vi "Auto Shift Control.vi"(11 "High/Low Gear Shift":bool) -> (3 "Low/High Gear Shift":enum16{"Off", "On", "Forward", "Reverse"}(ring))   [LabVIEW 2016]
uses:
  Global Variables/Low Gear Calibrations.vi
  Global Variables/Robot Status.vi
  Global Variables/Refnum Names.vi
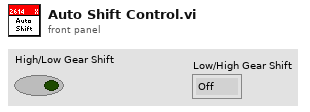
[diagram p1: front panel]
types:
  T1 = typedef "WPI_MotorControlDeviceRef.ctl" = cluster{"DeviceStatus":errorcluster, "Type":T2, "PWM":cluster{"PWM Channel":T3, "DeadBand":T4}, "CAN":cluster{"Device Number":u8, "SetOutput VI Ref":variant, "GetOutput VI Ref":variant, "Enable VI Ref":variant, "Disable VI Ref":variant, "Data":variant}, "Invert":bool}
  T2 = typedef "WPI_MotorControlType.ctl" = enum16{"PWM", "CAN"}
  T3 = typedef "FPGA_DIOPWMChannel.ctl" = enum8{"PWM 0", "PWM 1", "PWM 2", "PWM 3", "PWM 4", "PWM 5", "PWM 6", "PWM 7", "PWM 8", "PWM 9", "PWM MXP 0", "PWM MXP 1", "PWM MXP 2", "PWM MXP 3", "PWM MXP 4", "PWM MXP 5", "PWM MXP 6", "PWM MXP 7", "PWM MXP 8", "PWM MXP 9", "Invalid"}
  T4 = typedef "WPI_PWMDeadband.ctl" = cluster{"Name":string, "maxPositivePwm":i32, "minPositivePwm":i32, "centerPwm":i32, "maxNegativePwm":i32, "minNegativePwm":i32, "angularRange":u16}
  T5 = typedef "WPI_CANTalonSRX_GlobalStatus.ctl" = cluster{"Applied Throttle":dbl, "Module Enabled":bool, "CAN Error":errorcluster, "Closed Loop Error":dbl, "Forward Limit Switch Closed":bool, "Reverse Limit Switch Closed":bool, "Sensor Position":dbl, "Sensor Velocity":dbl, "Current":dbl, "Sticky Fault - Over Temp":bool, "Sticky Fault - Under Voltage":bool, "Sticky Fault - Forward Limit":bool, "Sticky Fault - Reverse Limit":bool, "Sticky Fault - Forward Soft Limit":bool, "Sticky Fault - Reverse Soft Limit":bool, "Brake is Enabled":bool, "Encoder Position":dbl, "Encoder Velocity":dbl, "Encoder Index Count":dbl, "Encoder A Pin State":bool, "Encoder B Pin State":bool, "Encoder Index Pin State":bool, "Analog In":dbl, "Analog In Velocity":dbl, "Temperature (C)":dbl, "Battery Voltage":dbl, "Control 5 Is Supported":bool, "Current Profile Slot Select":dbl, "Pos Div 8":bool, "Vel Div 4":bool, "Pulse Width Position":i32, "Pulse Width Velocity":i32, "Pulse Width Rise To Rise (us)":i32, "Pulse Width Rise To Fall (us)":i32, "Mot Prof Active Is Under Run":bool, "Mot Prof Active Has Under Run":bool, "Mot Prof Active Is Last":bool, "Mot Prof Active Velocity Only":bool, "Mot Prof Active Is Valid":bool, "Mot Prof Buffer Is Full":bool, "Mot Prof Active Profile Slot Select":i32, "Mot Prof NextID":i32, "Mot Prof Count":i32, "Mot Prof Active Velocity":dbl, "Mot Prof Active Position":dbl, "Mot Prof Output Enable":i32, "UsageFrame":u32, "Motion Magic Active Trajectory":cluster{"Velocity":dbl, "Position":dbl}}
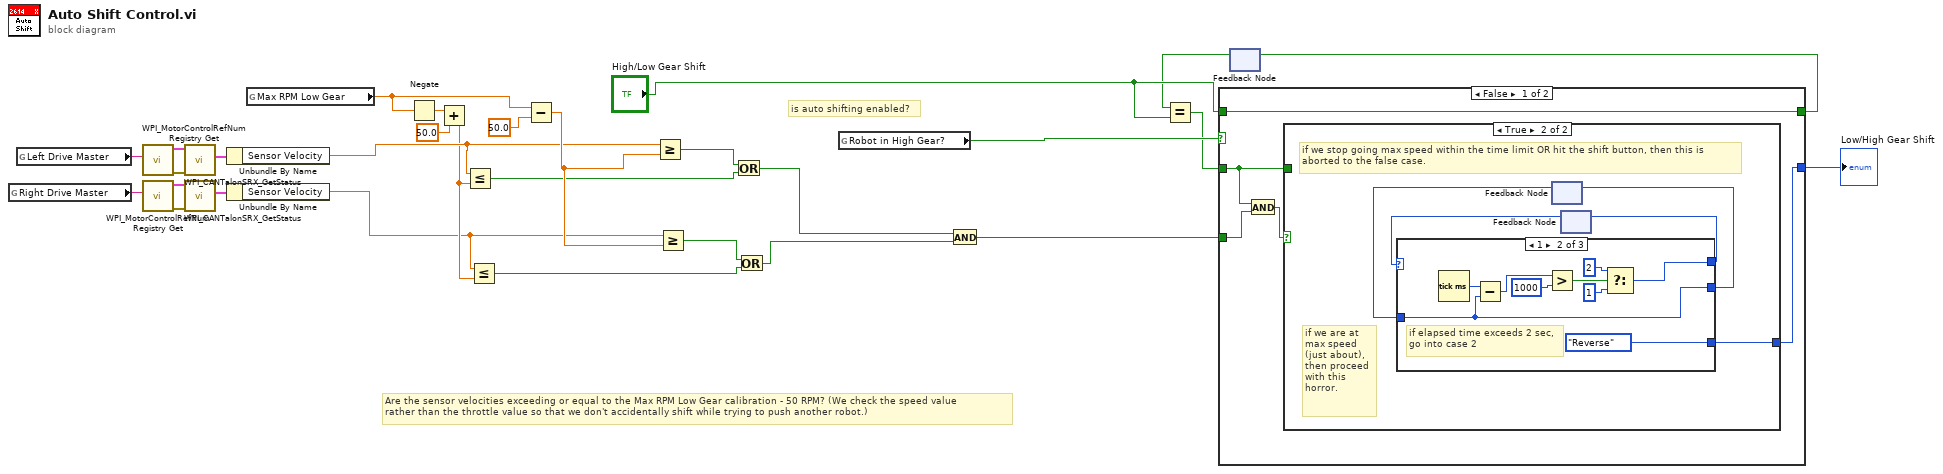
[diagram p0: block diagram]
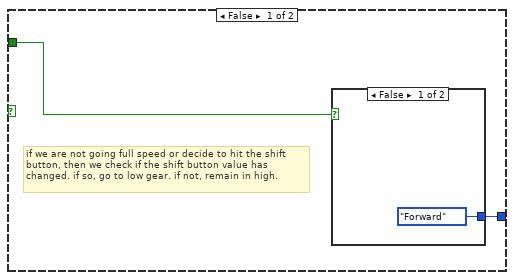
[diagram p2: hidden frame]
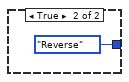
[diagram p3: hidden frame]
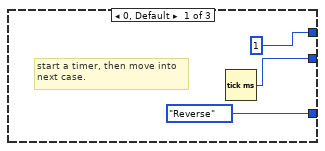
[diagram p4: hidden frame]
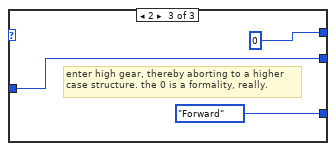
[diagram p5: hidden frame]
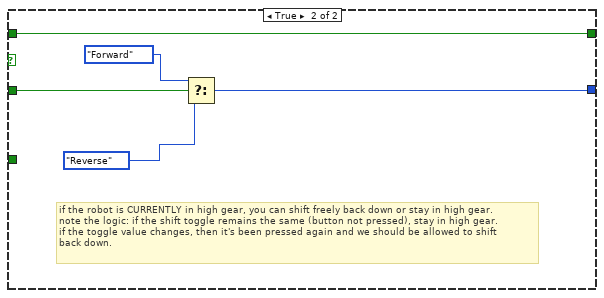
[diagram p6: hidden frame]
diagram:
  # "Are the sensor velocities exceeding or equal to the Max RPM Low Gear calibration - 50 RPM? (We check the speed value\nrather than the throttle value so that we don't accidentally shift while trying to push another robot.)"
  # "is auto shifting enabled?"
  n1 = global read "Refnum Names.vi" "Right Drive Master"() -> (w19:string)
  n2 = global read "Refnum Names.vi" "Left Drive Master"() -> (w22:string)
  n3 = call <vilib>:"WPI_MotorControlRefNum Registry Get.vi"("refnum name"=w22) -> ("error out"=w24:errorcluster, "MotorControlDevRef"=w23:T1)  [unwired: 9 in]
  n4 = call <vilib>:"WPI_MotorControlRefNum Registry Get.vi"("refnum name"=w19) -> ("error out"=w17:errorcluster, "MotorControlDevRef"=w18:T1)  [unwired: 9 in]
  n5 = call <vilib>:"WPI_CANTalonSRX_GetStatus.vi"("error in (no error)"=w24, "CAN Talon SRX Ref"=w23) -> ("Talon SRX Status"=w21:T5)  [unwired: 7 in, 2 out]
  n6 = call <vilib>:"WPI_CANTalonSRX_GetStatus.vi"("error in (no error)"=w17, "CAN Talon SRX Ref"=w18) -> ("Talon SRX Status"=w20:T5)  [unwired: 7 in, 2 out]
  n7 = Unbundle By Name(w21) -> ("Sensor Velocity"=w13:dbl)
  n8 = Unbundle By Name(w20) -> ("Sensor Velocity"=w11:dbl)
  n9 = global read "Low Gear Calibrations.vi" "Max RPM Low Gear"() -> (w16:dbl)
  n10 = Negate(x=w16) -> (-x=w14:dbl)
  n11 = Add(x=w14, y=50.0) -> (x+y=w12:dbl)
  n12 = Less Or Equal?(x=w13, y=w12) -> (x <= y?=w7:bool)
  n13 = Less Or Equal?(x=w11, y=w12) -> (x <= y?=w9:bool)
  n14 = Subtract(x=w16, y=50.0) -> (x-y=w25:dbl)
  n15 = Greater Or Equal?(x=w13, y=w25) -> (x >= y?=w8:bool)
  n16 = Greater Or Equal?(x=w11, y=w25) -> (x >= y?=w10:bool)
  n17 = Or(x=w8, y=w7) -> (x .or. y?=w6:bool)
  n18 = Or(x=w10, y=w9) -> (x .or. y?=w5:bool)
  n19 = global read "Robot Status.vi" "Robot in High Gear?"() -> (w28:bool)
  n20 = And(x=w6, y=w5) -> (x .and. y?=w27:bool)
  n21 = feedback #1() -> (w2:bool)  [unwired: 1 in]
  n22 = Equal?(x=w2, y="High/Low Gear Shift") -> (x = y?=w1:bool)
  n23 = case shown="False" w28 {
    tunnel: [w34 w59] -> w29
    tunnel: [w33 w63] -> w3
    tunnel: "High/Low Gear Shift" -> [w33 w63]
    tunnel: w1 -> [w32 w62]
    tunnel: w27 -> [w31 _]
    frame False {
      n24 = And(x=w32, y=w31) -> (x .and. y?=w30:bool)
      n25 = case shown="True" w30 {
        tunnel: [w36 w43] -> w34
        tunnel: w32 -> [w35 _]
        frame False {
          # "if we are not going full speed or decide to hit the shift\nbutton, then we check if the shift button value has\nchanged. if so, go to low gear. if not, remain in high."
          n26 = case shown="False" w35 {
            tunnel: [enum16{"Off", "On", "Forward", "Reverse"}."Forward" ("Low/High Gear Shift") enum16{"Off", "On", "Forward", "Reverse"}."Reverse" ("Low/High Gear Shift")] -> w36
            frame False {
            }
            frame True {
            }
          }
        }
        frame True {
          # "if we stop going max speed within the time limit OR hit the shift button, then this is\naborted to the false case."
          # "if we are at\nmax speed\n(just about),\nthen proceed\nwith this\nhorror."
          n27 = feedback #2() -> (w41:u32)  [unwired: 1 in]
          n28 = feedback #3() -> (w39:i32)  [unwired: 1 in]
          n29 = case shown="1" w39 {
            tunnel: [w46 w48 w57] -> w42
            tunnel: w41 -> [_ w48 w57]
            tunnel: [1 w49 0] -> w40
            tunnel: [enum16{"Off", "On", "Forward", "Reverse"}."Reverse" ("Low/High Gear Shift") enum16{"Off", "On", "Forward", "Reverse"}."Reverse" ("Low/High Gear Shift") enum16{"Off", "On", "Forward", "Reverse"}."Forward" ("Low/High Gear Shift")] -> w43
            frame 0, Default {
              # "start a timer, then move into\nnext case."
              n30 = Tick Count (ms)() -> (millisecond timer value=w46:u32)
            }
            frame 1 {
              # "if elapsed time exceeds 2 sec,\ngo into case 2"
              n31 = Tick Count (ms)() -> (millisecond timer value=w55:u32)
              n32 = Subtract(x=w55, y=w48) -> (x-y=w54:u32)
              n33 = Greater?(x=w54, y=u32 1000) -> (0:w52:bool)
              n34 = Select(t=2, s=w52, f=1) -> (s? t:f=w49:i32)
            }
            frame 2 {
              # "enter high gear, thereby aborting to a higher\ncase structure. the 0 is a formality, really."
            }
          }
          n35 = feedback-in #2(w42) -> ()
          n36 = feedback-in #3(w40) -> ()
        }
      }
    }
    frame True {
      # "if the robot is CURRENTLY in high gear, you can shift freely back down or stay in high gear.\nnote the logic: if the shift toggle remains the same (button not pressed), stay in high gear.\nif the toggle value changes, then it's been pressed again and we should be allowed to shift\nback down."
      n37 = Select(t=enum16{"Off", "On", "Forward", "Reverse"}."Forward" ("Low/High Gear Shift"), s=w62, f=enum16{"Off", "On", "Forward", "Reverse"}."Reverse" ("Low/High Gear Shift")) -> (s? t:f=w59:enum16{"Off", "On", "Forward", "Reverse"})
    }
  }
  "Low/High Gear Shift" <- w29
  n38 = feedback-in #1(w3) -> ()
